vi "Set Data Name.vi"(8 "error in (no error)":errorcluster, 10 "Data Name":string, 11 "LVData in":refnum<class "LVData.lvclass">) -> (0 "error out":errorcluster, 3 "LVData out":refnum<class "LVData.lvclass">)   [LabVIEW 2020, in "lvdata.lvlib" / "LVData.lvclass"]
uses:
  LVData.lvclass
  LVData.lvclass/LVData.ctl
  Bytes/Bytes.lvclass/Bytes.ctl
  02c30040-b776-42d1-95d1-d2856b7fa5f3.vi
  10f36b6c-deb1-498b-946e-e90237428c77.vi
  99d645ac-62e6-4010-a5fb-1574af8cd2a0.vi
  4a7d12f4-c3e6-4f69-80c0-5474c0967fdd.vi
  e692515c-7faf-4772-95d9-8d0673324605.vi
  ff636cc0-bfb6-4b84-88d0-e9252877989f.vi
  Type Descriptor/get_num_elements.vi/b3898c1b-5169-4cb1-894b-457c92b4a1c3.vi
  02c30040-b776-42d1-95d1-d2856b7fa5f3.vi/81433c74-ee36-47cf-a886-10c868675b30.vi
  02c30040-b776-42d1-95d1-d2856b7fa5f3.vi/d8d9ff34-2c15-4edb-a5ad-7260f11560db.vi
  Bytes/read.vi
  10f36b6c-deb1-498b-946e-e90237428c77.vi/9518bad7-5904-4cfc-9920-07fa30b29b3b.vi
  Bytes/to_data.vi
  99d645ac-62e6-4010-a5fb-1574af8cd2a0.vi/81433c74-ee36-47cf-a886-10c868675b30.vi
  99d645ac-62e6-4010-a5fb-1574af8cd2a0.vi/d8d9ff34-2c15-4edb-a5ad-7260f11560db.vi
  4a7d12f4-c3e6-4f69-80c0-5474c0967fdd.vi/92496872-6d84-4c82-887a-3ec8f8576b7c.vi
  Bytes/replace_bytes.vi
  e692515c-7faf-4772-95d9-8d0673324605.vi/92496872-6d84-4c82-887a-3ec8f8576b7c.vi
  ff636cc0-bfb6-4b84-88d0-e9252877989f.vi/92496872-6d84-4c82-887a-3ec8f8576b7c.vi
  Type Descriptor/get_num_elements.vi/b3898c1b-5169-4cb1-894b-457c92b4a1c3.vi/81433c74-ee36-47cf-a886-10c868675b30.vi
  Type Descriptor/get_num_elements.vi/b3898c1b-5169-4cb1-894b-457c92b4a1c3.vi/d8d9ff34-2c15-4edb-a5ad-7260f11560db.vi
  Bytes/from_byte_array.vi
  e692515c-7faf-4772-95d9-8d0673324605.vi/92496872-6d84-4c82-887a-3ec8f8576b7c.vi/2789ceee-8a64-4e3a-afcc-74e0c535c50e.vi
  Type Descriptor/TypeDescriptor.lvclass
  C:/projects/OpenG-Variant-Data-Library/source/library/Bytes/Bytes.lvclass
  read_type_descriptor.vi
  Bytes/Bytes.lvclass
  openg_variant.lvlib
  <userlib>/_OpenG.lib/error/error.llb/openg_error.lvlib
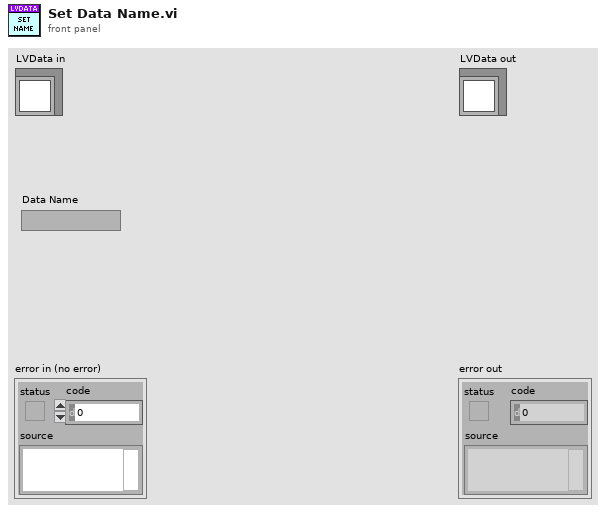
[diagram p1: front panel]
types:
  T1 = typedef "openg_variant.lvlib/Type Descriptor Enumeration.ctl" = enum8{"<Null>", "I8", "I16", "I32", "I64", "U8", "U16", "U32", "U64", "SGL", "DBL", "EXT", "CSG", "CDB", "CXT", "0x0F", "0x10", "0x11", "0x12", "0x13", "0x14", "Enum U8", "Enum U16", "Enum U32", "Enum U64", "SGL PQ", "DBL PQ", "EXT PQ", "CSG PQ", "CDB PQ", "CXT PQ", "0x1F", "0x20", "Boolean", "0x22", "0x23", "0x24", "0x25", "0x26", "0x27", "0x28", "0x29", "0x2A", "0x2B", "0x2C", "0x2D", "0x2E", "0x2F", "String", "0x31", "Path", "Pict", "0x34", "0x35", "0x36", "DAQ", "0x38", "0x39", "0x3A", "0x3B", "0x3C", "0x3D", "0x3E", "0x3F", "Array", "0x41", "0x42", "0x43", "0x44", "0x45", "0x46", "0x47", "0x48", "0x49", "0x4A", "0x4B", "0x4C", "0x4D", "0x4E", "0x4F", "Cluster", "0x51", "0x52", "Variant", "Waveform", "0x55", "0x56", "0x57", "0x58", "0x59", "0x5A", "0x5B", "0x5C", "0x5D", "0x5E", "Fixed Point", "0x60", "0x61", "0x62", "0x63", "0x64", "0x65", "0x66", "0x67", "0x68", "0x69", "0x6A", "0x6B", "0x6C", "0x6D", "0x6E", "0x6F", "Refnum", "0x71", "0x72", "Set Collection", "Map Collection"}
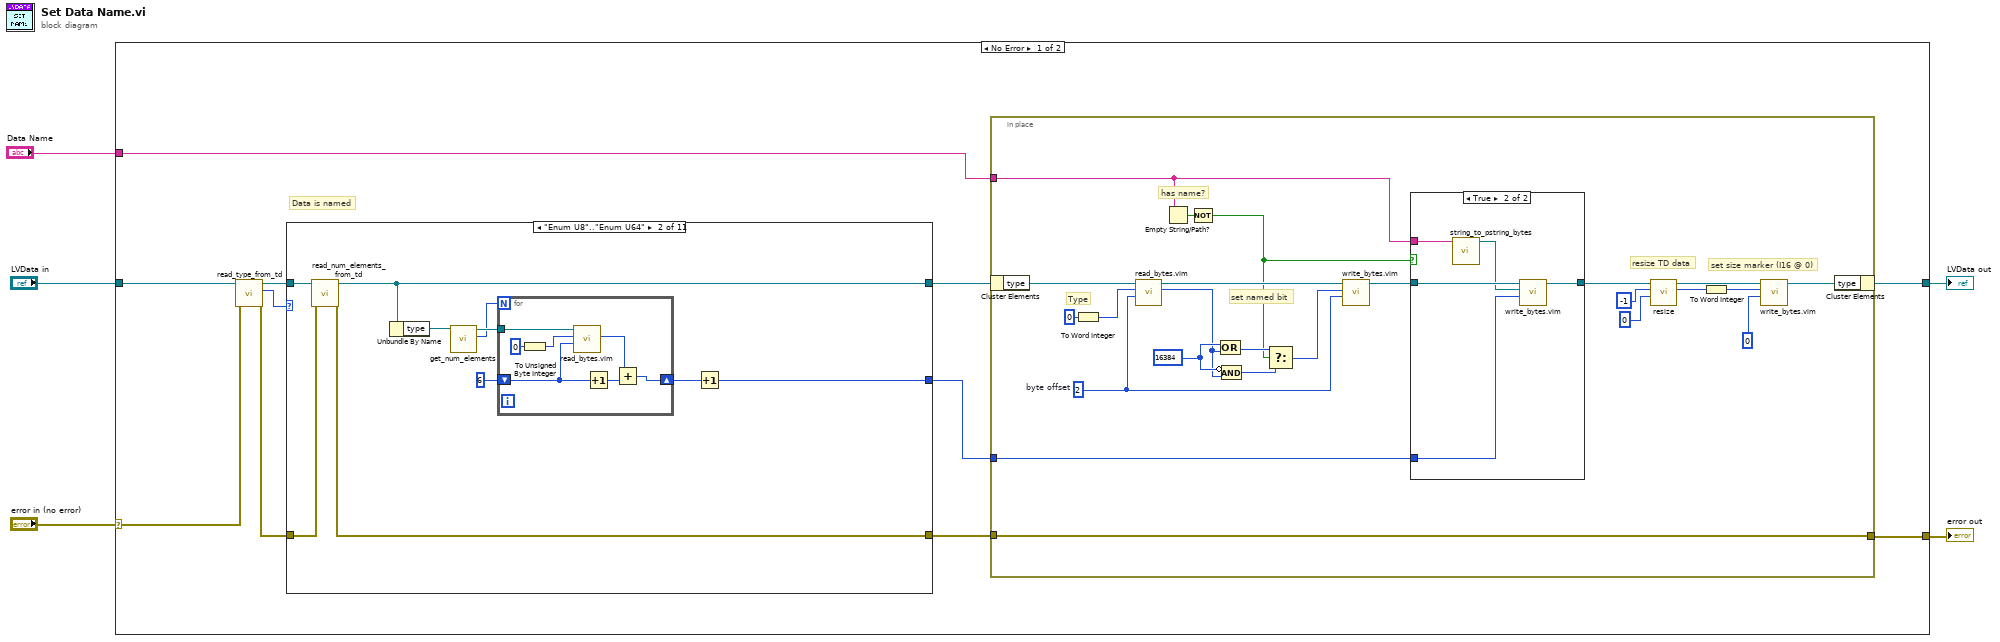
[diagram p0: block diagram]
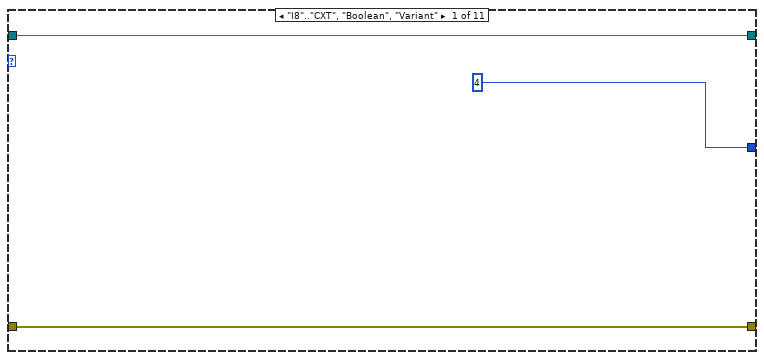
[diagram p2: hidden frame]
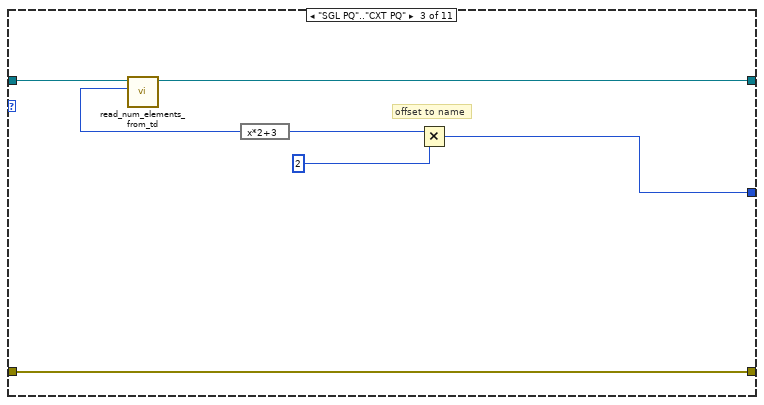
[diagram p3: hidden frame]
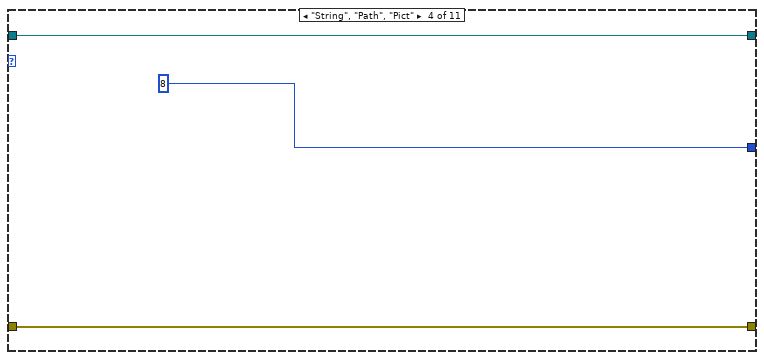
[diagram p4: hidden frame]
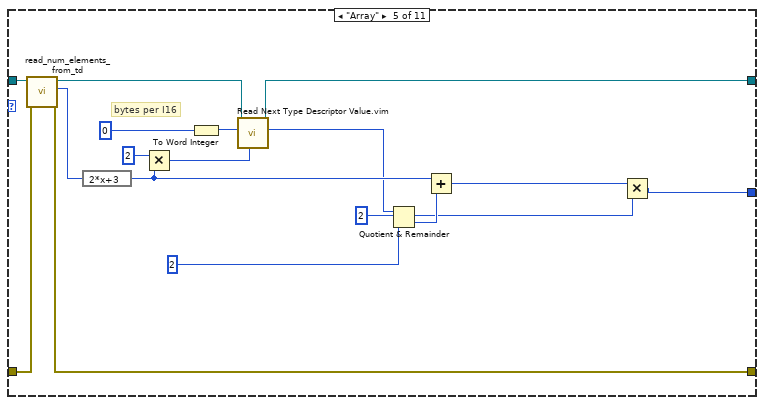
[diagram p5: hidden frame]
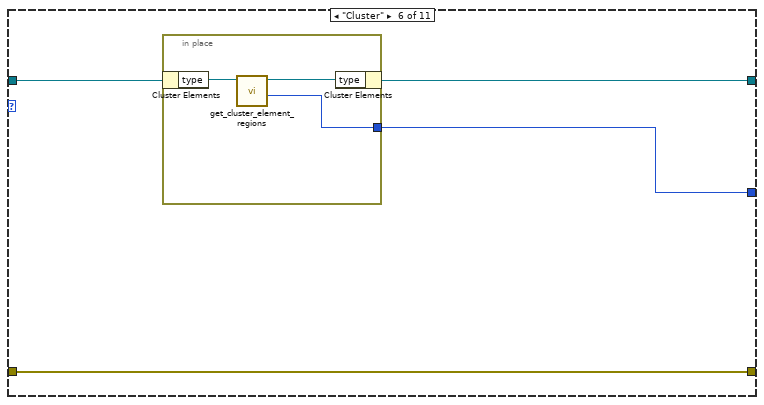
[diagram p6: hidden frame]
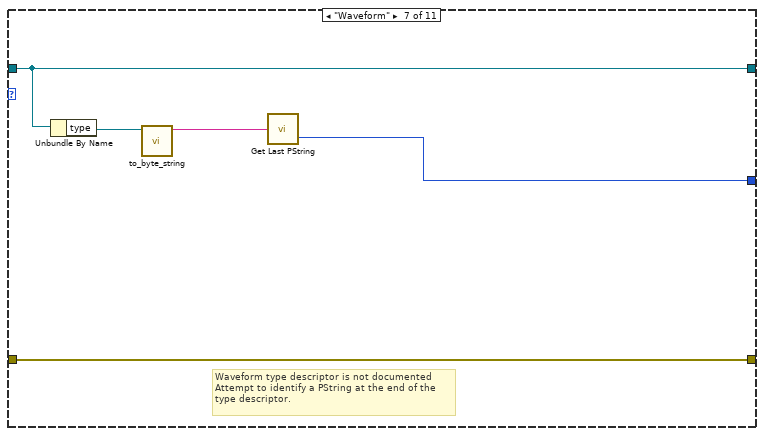
[diagram p7: hidden frame]
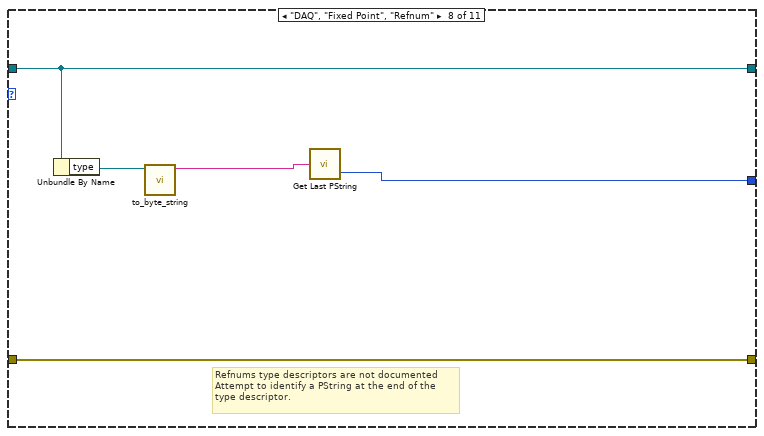
[diagram p8: hidden frame]
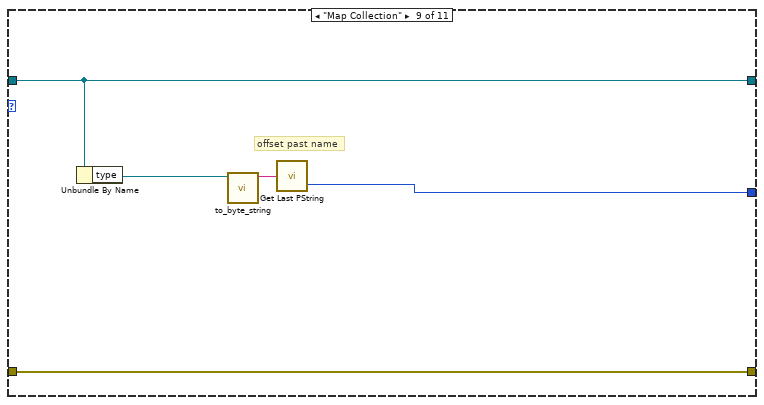
[diagram p9: hidden frame]
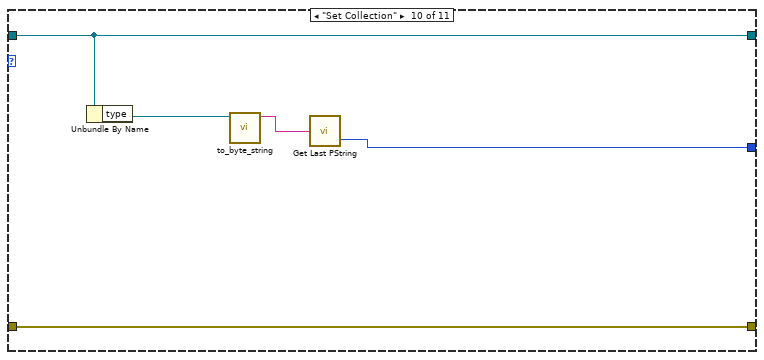
[diagram p10: hidden frame]
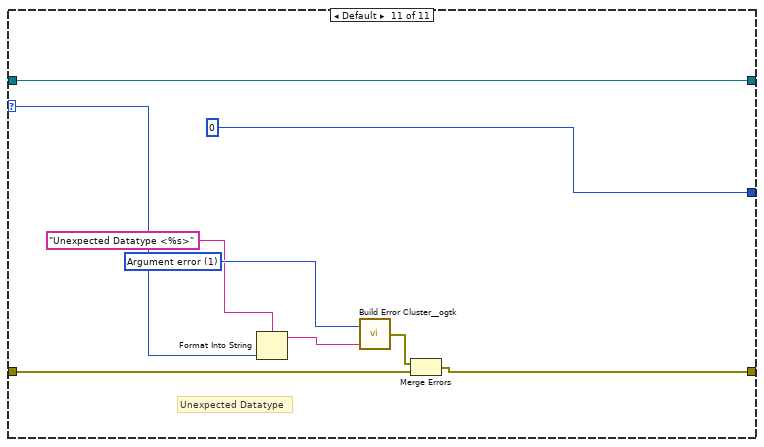
[diagram p11: hidden frame]
diagram:
  n1 = case shown="No Error" "error in (no error)" {
    selector: "error in (no error)" -> [w13 w131]
    tunnel: [w7 w131] -> w4
    tunnel: [w10 w130] -> w2
    tunnel: "LVData in" -> [w12 w130]
    tunnel: "Data Name" -> [w9 _]
    frame No Error {
      # "Data is named"
      n2 = call "read_type_from_td.vi"("error in (no error)"=w13, "LVData in"=w12) -> ("error out"=w14:errorcluster, "type"=w16:T1, "LVData out"=w15:refnum<class "LVData.lvclass">)  [unwired: 7 in]
      n3 = case shown="\"Enum U8\"..\"Enum U64\"" w16 {
        selector: w16 -> [_ _ _ _ _ _ _ _ _ _ w97]
        tunnel: [w19 w25 w43 w46 w59 w67 w75 w80 w85 w90 w93] -> w8
        tunnel: w14 -> [w19 w24 w43 w46 w58 w67 w75 w80 w85 w90 w95]
        tunnel: w15 -> [w18 w26 w41 w45 w61 w66 w73 w78 w83 w88 w92]
        tunnel: [w18 w27 w42 w45 w54 w64 w73 w78 w83 w88 w92] -> w11
        tunnel: [4 ("offset (0)") w23 w37 8 ("offset (0)") w47 w65 w71 w76 w81 w86 0 ("PString Offset")] -> w6
        frame "I8".."CXT", "Boolean", "Variant" {
        }
        frame "Enum U8".."Enum U64" {
          n4 = call "read_num_elements_from_td.vi"("error in (no error)"=w24, "LVData in"=w26) -> ("error out"=w25:errorcluster, "LVData out"=w27:refnum<class "LVData.lvclass">)  [unwired: 7 in, 1 out]
          n5 = Unbundle By Name(w27) -> ("type"=w22:refnum<class "TypeDescriptor.lvclass">)
          n6 = call "get_num_elements.vi"("TypeDescriptor"=w22) -> ("num_element"=w20:i32, "TypeDescriptor out"=w21:refnum<class "TypeDescriptor.lvclass">)  [unwired: 9 in]
          n7 = for {
            N: w20 -> [_]
            shift-right: [w30] -> w28
            shift-left: 6 -> [w33]
            tunnel: w21 -> [w36]
            n8 = To Unsigned Byte Integer(number=u8 0) -> (unsigned 8bit integer=w34:u8)
            n9 = call "read_bytes.vim"("byte offset"=w33, "data type"=w34, "Bytes in"=w36) -> ("value"=w31:u8)  [unwired: 7 in, 1 out]
            n10 = Increment(x=w33) -> (x+1=w32:i32)
            n11 = Add(x=w31, y=w32) -> (x+y=w30:i32)
          }
          n12 = Increment(x=w28) -> (x+1=w23:i32)
        }
        frame "SGL PQ".."CXT PQ" {
          # "offset to name"
          n13 = call "read_num_elements_from_td.vi"("LVData in"=w41) -> ("# elements"=w40:u16, "LVData out"=w42:refnum<class "LVData.lvclass">)  [unwired: 8 in, 1 out]
          n14 = expression code="x*2+3"(w40) -> (w38:u16)
          n15 = Multiply(x=w38, y=2) -> (x*y=w37:i32)
        }
        frame "String", "Path", "Pict" {
        }
        frame "Array" {
          # "bytes per I16"
          n16 = call "read_num_elements_from_td.vi"("error in (no error)"=w58, "LVData in"=w61) -> ("error out"=w59:errorcluster, "# elements"=w60:u16, "LVData out"=w55:refnum<class "LVData.lvclass">)  [unwired: 7 in]
          n17 = expression code="2*x+3"(w60) -> (w53:u16)
          n18 = Multiply(x=u16 2 ("y"), y=w53) -> (x*y=w51:u16)
          n19 = To Word Integer(number=u16 0 ("# elements")) -> (16bit integer=w57:i16)
          n20 = call "Read Next Type Descriptor Value.vim"("offset (-1)"=w51, "type"=w57, "LVData in"=w55) -> ("value"=w50:i16, "LVData out"=w54:refnum<class "LVData.lvclass">)  [unwired: 6 in, 1 out]
          n21 = Quotient & Remainder(x=w50, y=u16 2) -> (floor(x/y)=w62:u16)  [unwired: 1 out]
          n22 = Add(x=w53, y=w62) -> (x+y=w48:u16)
          n23 = Multiply(x=w48, y=2) -> (x*y=w47:i32)
        }
        frame "Cluster" {
          n24 = in-place {
            in-place-border: [w68] -> w65
            n25 = in-place-cluster #1(w66) -> ("type"=w70:refnum<class "TypeDescriptor.lvclass">)
            n26 = call "get_cluster_element_regions.vi"("TypeDescriptor"=w70) -> ("offset past element TDs"=w68:i32, "TypeDescriptor out"=w69:refnum<class "TypeDescriptor.lvclass">)  [unwired: 8 in, 1 out]
            n27 = in-place-cluster #1("type"=w69) -> (w64:refnum<class "LVData.lvclass">)
          }
        }
        frame "Waveform" {
          # "Waveform type descriptor is not documented\nAttempt to identify a PString at the end of the\ntype descriptor."
          n28 = Unbundle By Name(w73) -> ("type"=w74:refnum<class "TypeDescriptor.lvclass">)
          n29 = call "to_byte_string.vi"("Bytes in"=w74) -> ("byte string"=w72:string)  [unwired: 10 in]
          n30 = call "Get Last PString.vi"("String"=w72) -> ("PString Offset"=w71:i32)  [unwired: 1 out]
        }
        frame "DAQ", "Fixed Point", "Refnum" {
          # "Refnums type descriptors are not documented\nAttempt to identify a PString at the end of the\ntype descriptor."
          n31 = Unbundle By Name(w78) -> ("type"=w79:refnum<class "TypeDescriptor.lvclass">)
          n32 = call "to_byte_string.vi"("Bytes in"=w79) -> ("byte string"=w77:string)  [unwired: 10 in]
          n33 = call "Get Last PString.vi"("String"=w77) -> ("PString Offset"=w76:i32)  [unwired: 1 out]
        }
        frame "Map Collection" {
          # "offset past name"
          n34 = Unbundle By Name(w83) -> ("type"=w84:refnum<class "TypeDescriptor.lvclass">)
          n35 = call "to_byte_string.vi"("Bytes in"=w84) -> ("byte string"=w82:string)  [unwired: 10 in]
          n36 = call "Get Last PString.vi"("String"=w82) -> ("PString Offset"=w81:i32)  [unwired: 1 out]
        }
        frame "Set Collection" {
          n37 = Unbundle By Name(w88) -> ("type"=w89:refnum<class "TypeDescriptor.lvclass">)
          n38 = call "to_byte_string.vi"("Bytes in"=w89) -> ("byte string"=w87:string)  [unwired: 10 in]
          n39 = call "Get Last PString.vi"("String"=w87) -> ("PString Offset"=w86:i32)  [unwired: 1 out]
        }
        frame Default {
          w99 = 1 items=["No error", "Argument error", "Memory is full", "Out of zone", "End of file", "File already open", "Generic file I/O error", "File not found", "File permission error", "Disk is full", "Duplicate path", "Too many files open", "System feature not enabled", "Resource file not found", "Cannot add resource", "Resource not found", "Image not found", "Image memory error", "Pen does not exist", "Config type invalid", "Config token not found", "Config parse error", "Config memory error", "Bad external code format", "Bad external code offset", "External code not present", "Null window", "Destroy window error", "Null menu", "Print aborted", "Bad print record", "Print driver error", "Windows error during printing", "Memory error during printing", "Print dialog error", "Generic print error", "Invalid device refnum", "Device not found", "Device parameter error", "Device unit error", "Cannot open device", "Device call aborted", "Generic error", "Cancelled by user", "Object ID too low", "Object ID too high", "Object not in heap", "Unknown heap", "Unknown object (invalid DefProc)", "Unknown object (DefProc not in table)", "Message out of range", "Invalid (null) method", "Unknown message", "Manager call not supported", "Bad address", "Network operation in progress", "Network operation timed out", "Connection is busy", "Network attribute not supported", "Network error", "Address in use", "System out of memory", "Connection aborted", "Connection refused", "Not connected", "Already connected", "Connection closed", "Initialization error (interapplication manager)", "Bad occurrence", "Wait on unbound occurrence handler", "Occurrence queue overflow", "Datalog type conflict", "Unused", "Unrecognized type (interapplication manager)", "Memory corrupt", "Failed to make temporary DLL", "Old CIN version", "Drag socket not found", "Failed to load drop-object", "Failed to register OLE object", "Failed to release OLE object", "Format specifier type mismatch", "Unknown format specifier", "Too few format specifiers", "Too many format specifiers", "Scan failed", "Newer CIN version", "Error converting to variant", "Runtime menu error", "Password tampered", "Variant attribute not found", "Incompatible variant data type", "Event data is not available", "Event Store is not present", "Occurrence is not found", "Event Queue is not created", "Event info is not available", "Refnum passed is NULL", "Error retrieving Class GUID", "Error retrieving CoClass GUID", "Error retrieving TypeLib GUID.", "Bad built application magic bytes.", "Specific driver is different from the specific driver associated with the Logical Name.", "There is no session opened to the class driver.", "Max Error", "MAX - Error with config objects", "MAX - Error loading configuration", "MAX - Group not supported"]
          # "Unexpected Datatype"
          n40 = Format Into String(format string="Unexpected Datatype <%s>" ("Format String"), w97) -> (resulting string=w96:string)  [unwired: 2 in, 1 out]
          n41 = call <userlib>:"Build Error Cluster__ogtk.vi"("String to Prepend to source (\"\")"=w96, "code"=w99) -> ("error out"=w94:errorcluster)
          n42 = Merge Errors(w94, w95) -> (w93:errorcluster)
        }
      }
      n43 = in-place {
        in-place-border: w9 -> [w113]
        in-place-border: w8 -> [w110]
        in-place-border: [w110] -> w7
        in-place-border: w6 -> [w109]
        w123 = i16 16384 ("Input")
        w100 = 2  # byte offset
        # "resize TD data"
        # "set size marker (I16 @ 0)"
        # "has name?"
        # "Type"
        # "set named bit"
        n44 = in-place-cluster #2(w11) -> ("type"=w111:refnum<class "TypeDescriptor.lvclass">)
        n45 = To Word Integer(number=i16 0) -> (16bit integer=w116:i16)
        n46 = call "read_bytes.vim"("byte offset"=w100, "data type"=w116, "Bytes in"=w111) -> ("value"=w119:i16, "Bytes out"=w118:refnum<class "TypeDescriptor.lvclass">)  [unwired: 7 in]
        n47 = Empty String/Path?(string/path=w113) -> (empty?=w114:bool)
        n48 = Not(x=w114) -> (.not. x?=w112:bool)
        n49 = Compound Arithmetic op=OR(w123, w119) -> (w122:i16)
        n50 = Compound Arithmetic op=AND(invert w123, w119) -> (w121:i16)
        n51 = Select(t=w122, s=w112, f=w121) -> (s? t:f=w117:i16)
        n52 = call "write_bytes.vim"("offset (-1: current position)"=w100, "value"=w117, "Bytes in"=w118) -> ("Bytes out"=w115:refnum<class "TypeDescriptor.lvclass">)  [unwired: 8 in]
        n53 = case shown="True" w112 {
          tunnel: w115 -> [w124 w129]
          tunnel: [w124 w128] -> w108
          tunnel: w113 -> [_ w126]
          tunnel: w109 -> [_ w125]
          frame False {
          }
          frame True {
            n54 = call "string_to_pstring_bytes.vi"("string"=w126) -> ("PString Bytes"=w127:refnum<class "Bytes.lvclass">)  [unwired: 10 in]
            n55 = call "write_bytes.vim"("offset (-1: current position)"=w125, "value"=w127, "Bytes in"=w129) -> ("Bytes out"=w128:refnum<class "TypeDescriptor.lvclass">)  [unwired: 8 in]
          }
        }
        n56 = call "resize.vi"("new_size (from offset)"=0, "offset (-1: current position)"=-1, "Bytes in"=w108) -> ("total_size"=w105:i32, "Bytes out"=w104:refnum<class "TypeDescriptor.lvclass">)  [unwired: 6 in, 1 out]
        n57 = To Word Integer(number=w105) -> (16bit integer=w101:i16)
        n58 = call "write_bytes.vim"("offset (-1: current position)"=0, "value"=w101, "Bytes in"=w104) -> ("Bytes out"=w103:refnum<class "TypeDescriptor.lvclass">)  [unwired: 8 in]
        n59 = in-place-cluster #2("type"=w103) -> (w10:refnum<class "LVData.lvclass">)
      }
    }
    frame Error {
    }
  }
  "error out" <- w4
  "LVData out" <- w2
